vi "MRB_get.vi"(8 "err_in":errorcluster, 11 "visa_in":refnum<visa-resource-name>) -> (0 "err_out":errorcluster, 2 "opening":dbl, 3 "visa_out":refnum<visa-resource-name>, 4 "status":bool)   [LabVIEW 2019]
panel:
  out "read count":u32
  out "write count":u32
  out "string":string
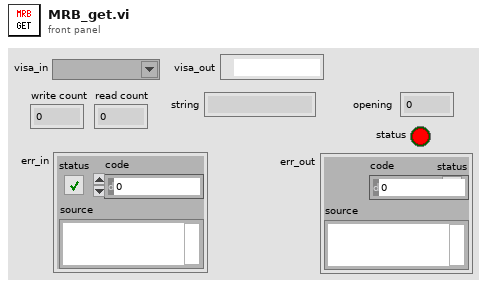
[diagram p1: front panel]
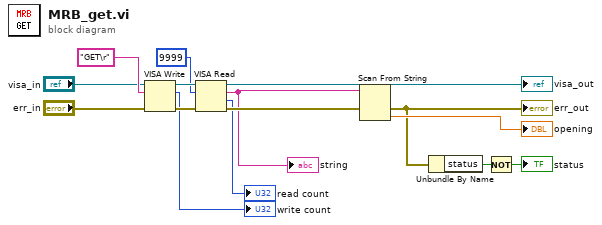
[diagram p0: block diagram]
diagram:
  n1 = VISA Write(VISA resource name="visa_in", write buffer="GET\r" ("string"), error in (no error)="err_in") -> (VISA resource name out=w15:refnum<visa-resource-name>, return count=→"write count":u32, error out=w14:errorcluster)
  n2 = VISA Read(VISA resource name=w15, byte count=u32 9999, error in (no error)=w14) -> (VISA resource name out=→"visa_out":refnum<visa-resource-name>, read buffer=w3:string, return count=→"read count":u32, error out=w7:errorcluster)
  "string" <- w3
  n3 = Scan From String(input string=w3, error in=w7) -> (error out=w6:errorcluster, output 1=→"opening":dbl)  [unwired: 3 in, 2 out]
  "err_out" <- w6
  n4 = Unbundle By Name(w6) -> ("status"=w5:bool)
  n5 = Not(x=w5) -> (.not. x?=→"status":bool)
